vi "Process.vi"(8 "error in":errorcluster, 11 "Plugin in":refnum<class "RPM Measurement.lvclass">) -> (0 "error out":errorcluster, 3 "Plugin out":refnum<class "RPM Measurement.lvclass">)   [LabVIEW 2020, in "RPM Measurement.lvlib" / "RPM Measurement.lvclass"]
uses:
  RPM Measurement.lvclass
  C:/Program Files/National Instruments/LabVIEW 2020/vi.lib/FlexLogger/SDK/PluginSDK.lvlibp/PEFClasses/SDK/Plugin/Plugin.lvclass
  RPM Measurement.lvclass/RPM Measurement.ctl
  <vilib>/FlexLogger/SDK/PluginSDK.lvlibp/PEFClasses/SDK/Plugin/DataHelpers/Write 1D Wfm (DBL).vi
  <vilib>/FlexLogger/SDK/PluginSDK.lvlibp/PEFClasses/SDK/Plugin/Plugin.lvclass
  C:/Program Files/National Instruments/LabVIEW 2020/vi.lib/FlexLogger/SDK/PluginSDK.lvlibp/PEFClasses/SDK/Processing Element/Processing Element.lvclass
  C:/Users/NIIndiaAE/Desktop/FlexLogger Plugin/RPM Plugin/RPM Measurement.lvclass
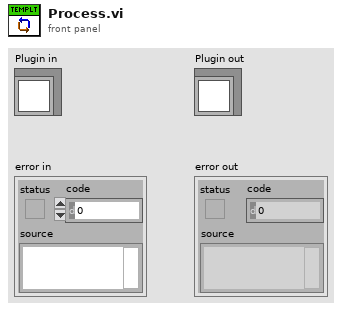
[diagram p1: front panel]
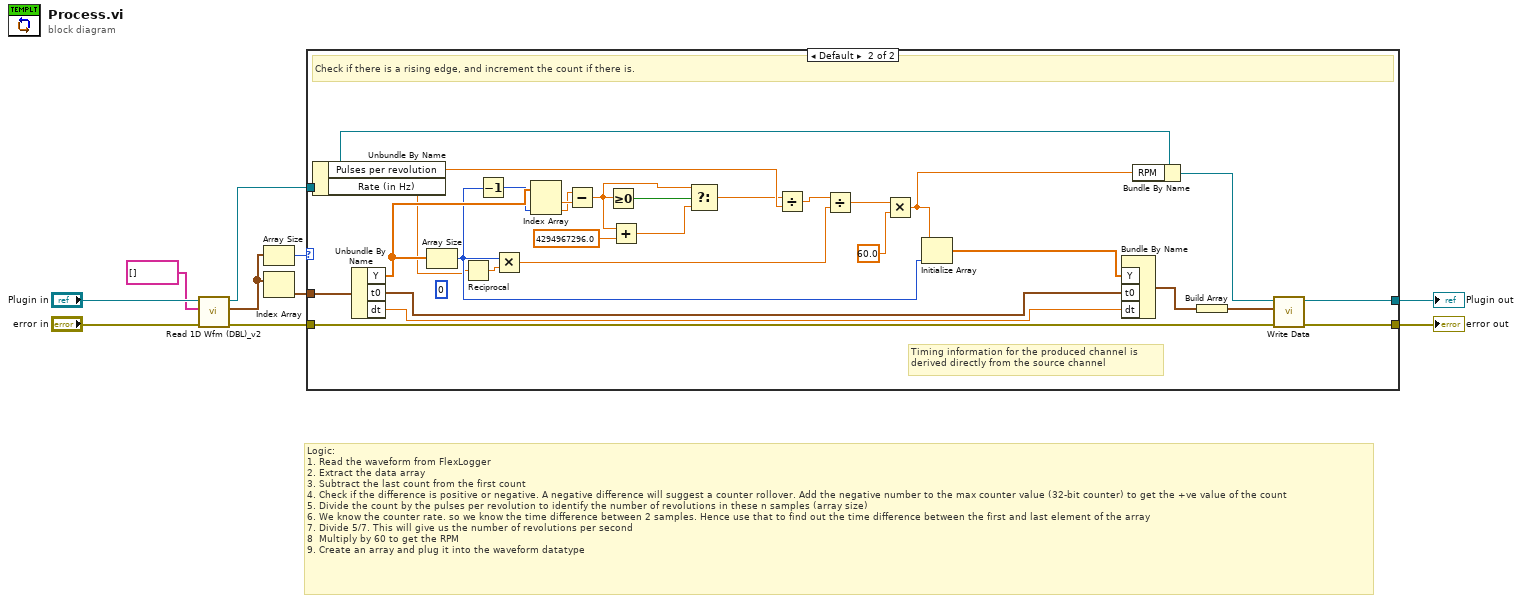
[diagram p0: block diagram]
diagram:
  # "Logic:\n1. Read the waveform from FlexLogger\n2. Extract the data array\n3. Subtract the last count from the first count\n4. Check if the difference is positive or negative. A negative difference will suggest a counter rollover. Add the negative number to the max counter value (32-bit counter) to get the +ve value of the count\n5. Divide the count by the pulses per revolution to identify the number of revolutions in these n samples (array size)\n6. We know the counter rate. so we know the time difference between 2 samples. Hence use that to find out the time difference between the first and last element of the array\n7. Divide 5/7. This will give us the number of revolutions per second\n8  Multiply by 60 to get the RPM\n9. Create an array and plug it into the waveform datatype"
  n1 = call <vilib>:"Read 1D Wfm (DBL)_v2.vi"("error in (no error)"="error in", "Unique Identifers (empty = all)"=string[] [] ("Unique Channel Identifers (empty = all)"), "Plugin in"="Plugin in") -> ("error out"=w4:errorcluster, "Data"=w2:waveform(dbl)[], "Plugin out"=w5:refnum<class "RPM Measurement.lvclass">)  [unwired: 5 in, 1 out]
  n2 = Array Size(array=w2) -> (size(s)=w6:i32)
  n3 = Index Array(array=w2) -> (element=w1:waveform(dbl))  [unwired: 1 in]
  n4 = case shown="Default" w6 {
    tunnel: w1 -> [_ w38]
    tunnel: [w11 w36] -> w8
    tunnel: [w12 w35] -> w7
    tunnel: w5 -> [w12 w33]
    tunnel: w4 -> [w11 w34]
    frame 0 {
      # "No channels sending data to the plugin"
    }
    frame Default {
      (unwired) 0 ("index")
      # "Timing information for the produced channel is\nderived directly from the source channel"
      # "Check if there is a rising edge, and increment the count if there is."
      n5 = Unbundle By Name(w33) -> ("Pulses per revolution"=w19:dbl, "Rate (in Hz)"=w22:dbl)
      n6 = Unbundle By Name(w38) -> ("Y"=w31:dbl[], "t0"=w40:timestamp, "dt"=w39:dbl)
      n7 = Array Size(array=w31) -> (size(s)=w23:i32)
      n8 = Reciprocal(x=w22) -> (1/x=w21:dbl)
      n9 = Decrement(x=w23) -> (x-1=w30:i32)
      n10 = Multiply(x=w23, y=w21) -> (x*y=w27:dbl)
      n11 = Index Array(array=w31, index #2=w30) -> (element #1=w29:dbl, element #2=w28:dbl)  [unwired: 1 in]
      n12 = Subtract(x=w28, y=w29) -> (x-y=w17:dbl)
      n13 = Greater Or Equal To 0?(x=w17) -> (x >= 0?=w18:bool)
      n14 = Add(x=w17, y=4294967296.0) -> (x+y=w15:dbl)
      n15 = Select(t=w17, s=w18, f=w15) -> (s? t:f=w14:dbl)
      n16 = Divide(x=w14, y=w19) -> (x/y=w20:dbl)
      n17 = Divide(x=w20, y=w27) -> (x/y=w26:dbl)
      n18 = Multiply(x=w26, y=60.0) -> (x*y=w24:dbl)
      n19 = Initialize Array(w24, w23) -> (w13:dbl[])
      n20 = Bundle By Name("Y"=w13, "t0"=w40, "dt"=w39) -> (w41:waveform(dbl))  [unwired: 1 in]
      n21 = Bundle By Name(cluster=w33, "RPM"=w24) -> (w32:refnum<class "RPM Measurement.lvclass">)
      n22 = Build Array(w41) -> (w37:waveform(dbl)[])
      n23 = call-poly <vilib>:"Write Data.vi"("error in (no error)"=w34, "Data"=w37, "Plugin in"=w32) -> ("error out"=w36:errorcluster, "Plugin out"=w35:refnum<class "RPM Measurement.lvclass">)  [unwired: 7 in]
    }
  }
  "error out" <- w8
  "Plugin out" <- w7
